vi "Measure.vi"(0 "Startfeld (T)":dbl=0.1, 1 "Zielfeld (T)":dbl=-0.1, 2 "Sweeprate (T/min)":dbl=0.05 min=0.0, 3 "Delay bei Null":bool=TRUE, 4 "Delay bei Max/Min":bool=TRUE, 5 "Delaytime bei Null (s)":u32=10, 6 "Anzahl Sweeps":u32=2, 7 "Deviation":u16(ring) items=["Normal", "Deviation"], 8 "Backsweep":bool=TRUE, 9 "Messmodus":u16(ring) items=["Nanosiemens", "Dissipation-tan(delta)", "Series - KilOhms", "GigOhms", "Loss Vector"], 10 "to Zero":bool=TRUE, 11 "error in (no error)":errorcluster) -> (14 "Ausgabe-Cluster":T1, 19 "error out":errorcluster)   [LabVIEW 2009]
panel:
  in  "Stop bei Target":bool
  out "Data":bool
  out "Done":bool
  in  "Delaytime bei Max/Min (s)":u32=10
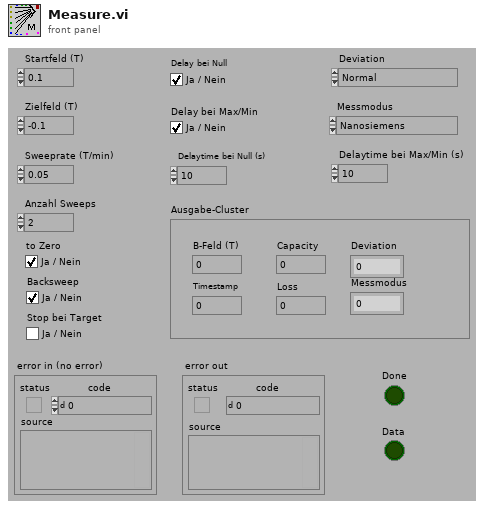
[diagram p1: front panel]
types:
  T1 = cluster{"B-Feld (T)":dbl, "Timestamp":dbl, "Capacity":dbl, "Loss":dbl, "Deviation":u16, "Messmodus":u16}
  T2 = cluster{"B-Feld":dbl, dbl, "capacitance":dbl, "loss":dbl, "Deviation":u16, "Messmodus":u16}
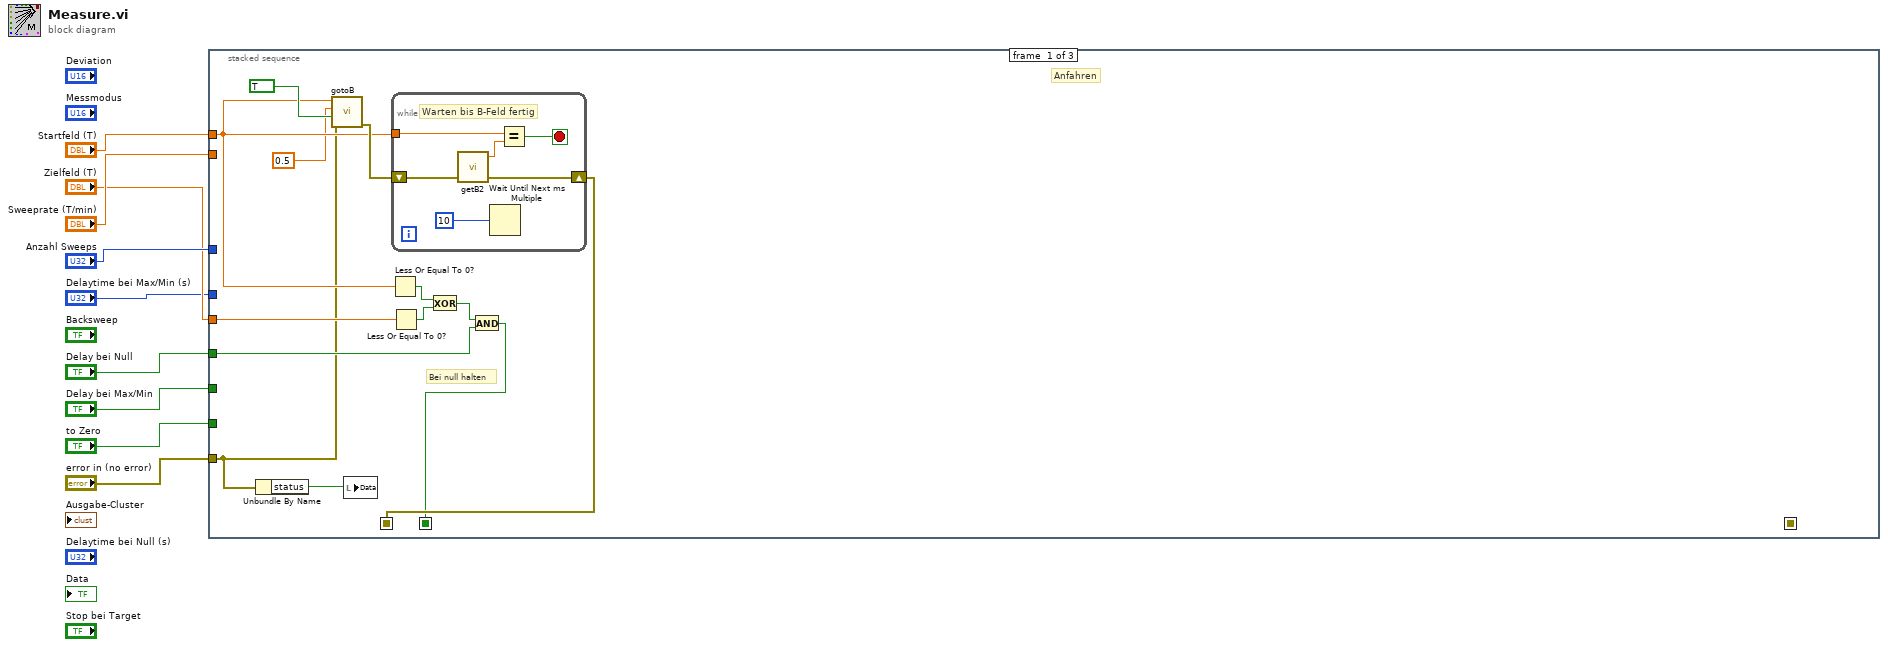
[diagram p0: block diagram]
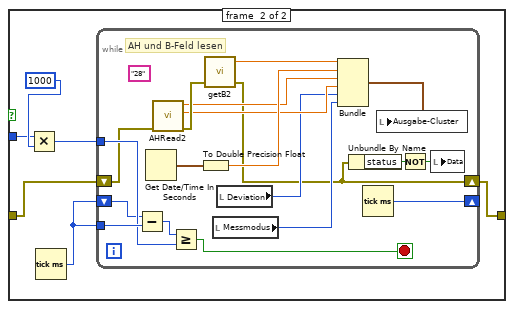
[diagram p3: hidden frame]
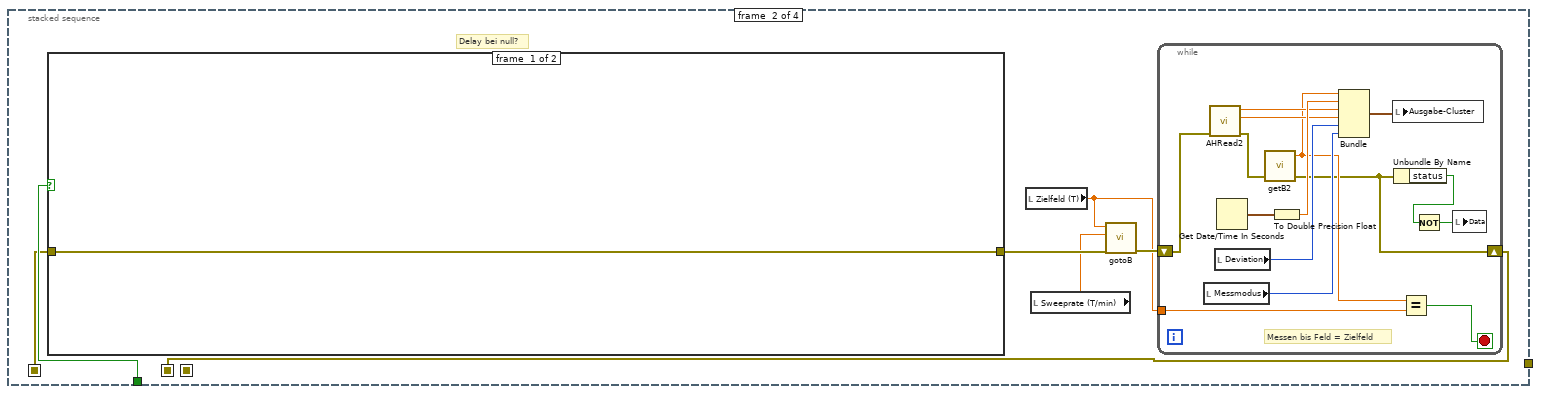
[diagram p4: hidden frame]
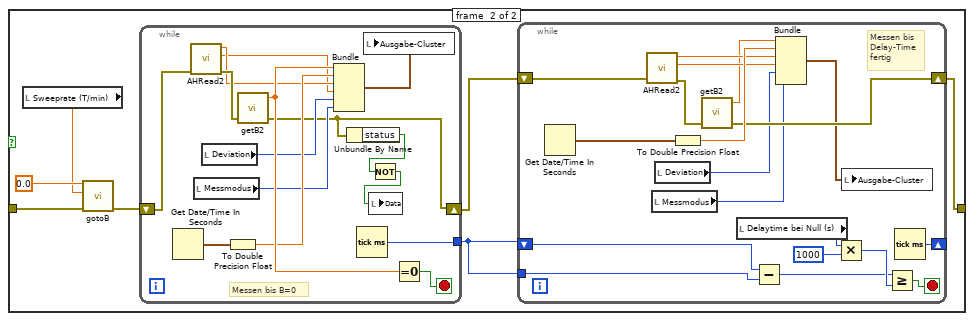
[diagram p5: hidden frame]
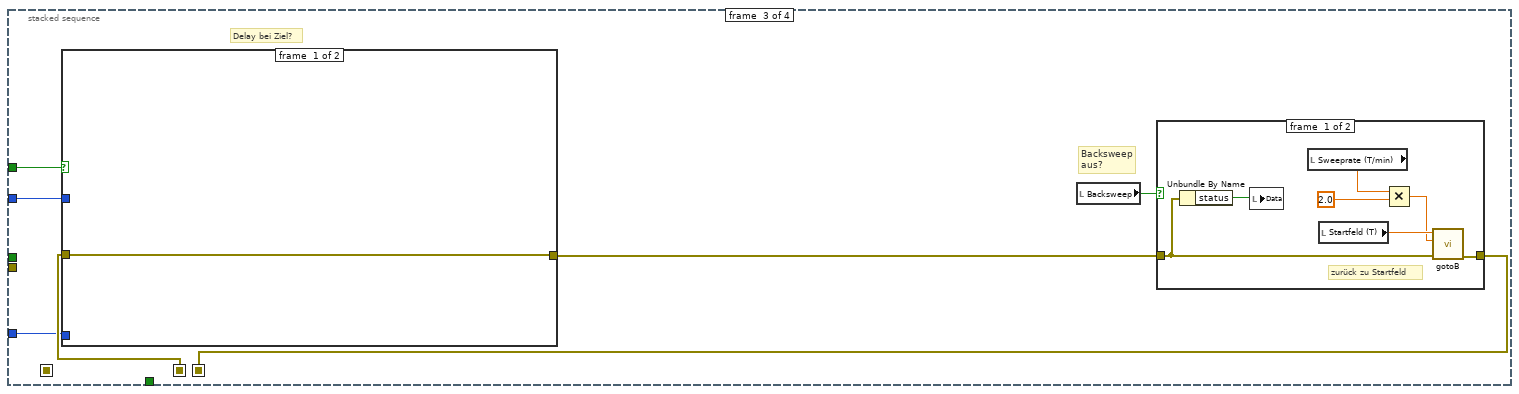
[diagram p6: hidden frame]
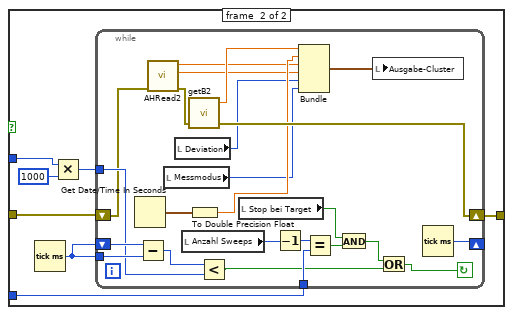
[diagram p8: hidden frame]
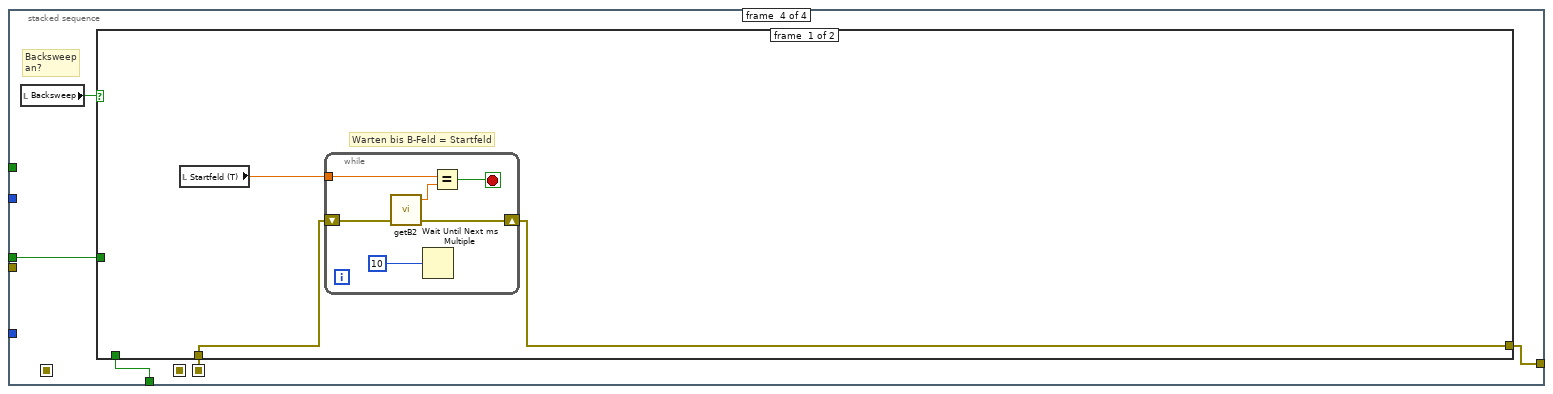
[diagram p9: hidden frame]
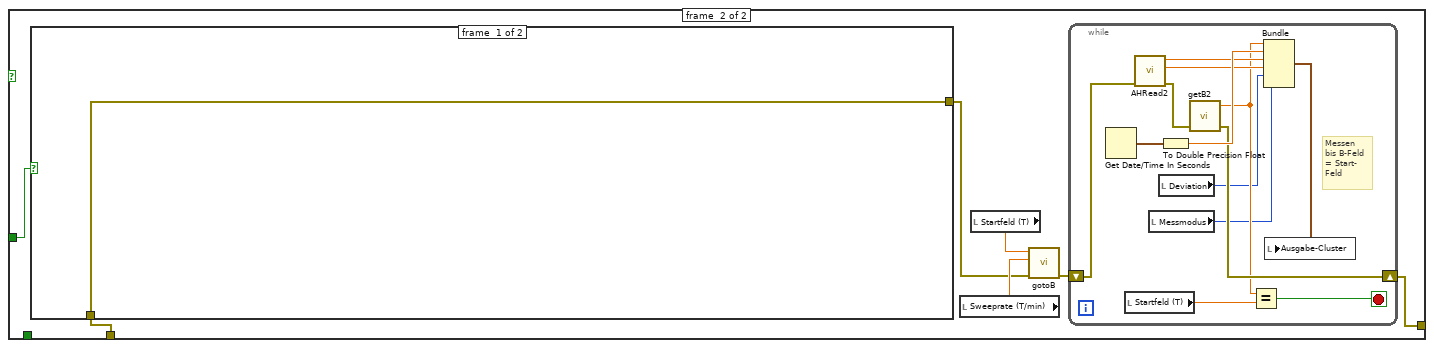
[diagram p10: hidden frame]
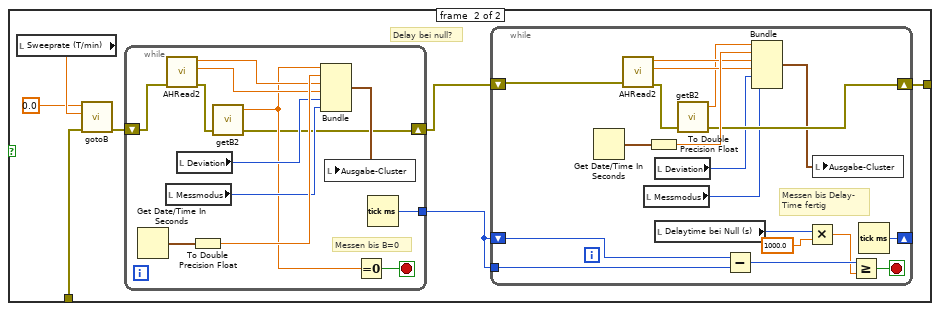
[diagram p11: hidden frame]
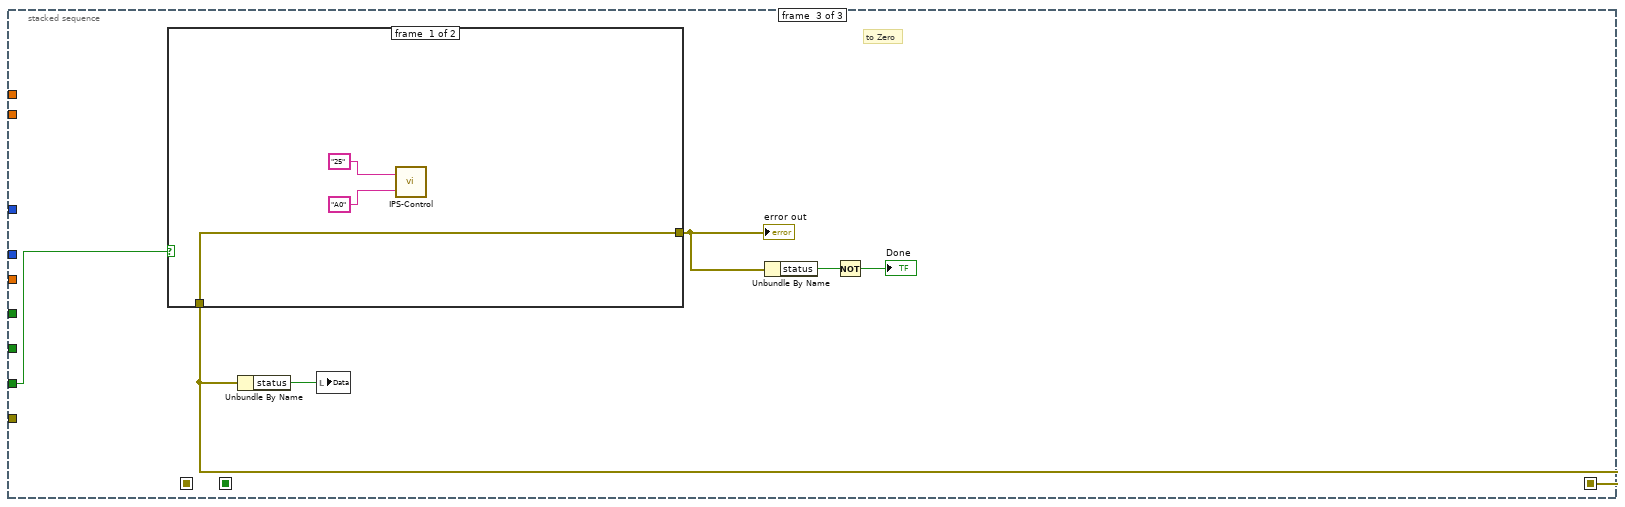
[diagram p12: hidden frame]
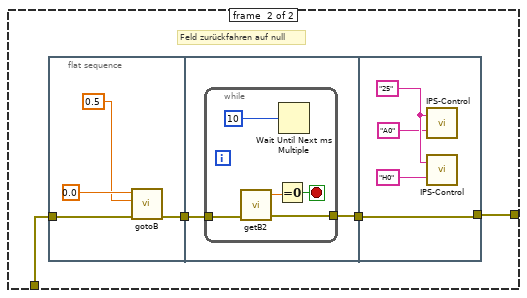
[diagram p13: hidden frame]
diagram:
  n1 = stacked-sequence {
    seq-local: [w20 _ _] -> [_ w36 _]
    seq-local: [w13 _ _] -> [_ w35 _]
    seq-local: [_ w30 _] -> [_ _ w261]
    tunnel: "Startfeld (T)" -> [w19 _ _]
    tunnel: "Sweeprate (T/min)" -> [_ w33 _]
    tunnel: "error in (no error)" -> [w12 _ _]
    tunnel: "Anzahl Sweeps" -> [_ w37 _]
    tunnel: "Zielfeld (T)" -> [w18 w34 _]
    tunnel: "Delay bei Null" -> [w14 w31 _]
    tunnel: "Delay bei Max/Min" -> [_ w32 _]
    tunnel: "to Zero" -> [_ _ w265]
    tunnel: "Delaytime bei Max/Min (s)" -> [_ w29 _]
    frame #0 {
      # "Bei null halten"
      # "Anfahren"
      n2 = Unbundle By Name(w12) -> ("status"=w11:bool)
      n3 = call "gotoB.vi"("error in (no error)"=w12, "Heater"=TRUE, "Sweeprate (T/min)"=0.5, "Target Field (T)"=w19) -> ("error out"=w21:errorcluster)  [unwired: 7 in]
      n4 = local write "Data"(w11) -> ()
      n5 = Less Or Equal To 0?(x=w19) -> (x <= 0?=w16:bool)
      n6 = Less Or Equal To 0?(x=w18) -> (x <= 0?=w17:bool)
      n7 = while {
        tunnel: w19 -> [w27]
        shift-right: [w25] -> w20
        shift-left: w21 -> [w26]
        stop <- w24 stop-if-true
        # "Warten bis B-Feld fertig"
        n8 = call "getB2.vi"("error in (no error)"=w26) -> ("error out"=w25:errorcluster, "B-Feld"=w28:dbl)  [unwired: 3 in]
        n9 = Wait Until Next ms Multiple(millisecond multiple=10) -> ()  [unwired: 1 out]
        n10 = Equal?(x=w27, y=w28) -> (x = y?=w24:bool)
      }
      n11 = Exclusive Or(1:w17, 2:w16) -> (0:w15:bool)
      n12 = And(x=w15, y=w14) -> (x .and. y?=w13:bool)
    }
    frame #1 {
      # "Wiederholung Anzahl Sweeps"
      # "Messung"
      n13 = for {
        N: w37 -> [_]
        shift-right: [w40] -> w30
        shift-left: w36 -> [w43]
        tunnel: w35 -> [w42]
        tunnel: w34 -> [_]
        tunnel: w33 -> [_]
        tunnel: w32 -> [w44]
        tunnel: w31 -> [w41]
        tunnel: w29 -> [w39]
        i -> [w38]
        n14 = stacked-sequence {
          seq-local: [w47 _ _ _] -> [_ w80 _ _]
          seq-local: [_ w75 _ _] -> [_ _ w144 _]
          seq-local: [_ _ w141 _] -> [_ _ _ w189]
          tunnel: w44 -> [w48 _ w145 _]
          tunnel: w43 -> [w45 _ _ _]
          tunnel: w42 -> [_ w81 _ w188]
          tunnel: w41 -> [_ _ _ w187]
          tunnel: [_ _ _ w186] -> w40
          tunnel: w39 -> [w46 _ w140 _]
          tunnel: w38 -> [_ _ w139 _]
          frame #0 {
            # "Delay bei Start?"
            n15 = case shown="True" w48 {
              tunnel: w45 -> [w49 w53]
              tunnel: [w49 w52] -> w47
              tunnel: w46 -> [_ w50]
              frame #0 {
              }
              frame #1 {
                n16 = Multiply(x=w50, y=1000) -> (x*y=w54:u32)
                n17 = Tick Count (ms)() -> (millisecond timer value=w51:u32)
                n18 = while {
                  tunnel: w51 -> [w74]
                  tunnel: w54 -> [w72]
                  shift-right: [w69] -> _
                  shift-left: w51 -> [w70]
                  shift-right: [w56] -> w52
                  shift-left: w53 -> [w68]
                  stop <- w71 stop-if-true
                  (unwired) "28"
                  # "AH und B-Feld lesen"
                  n19 = Subtract(x=w70, y=w74) -> (x-y=w73:u32)
                  n20 = Get Date/Time In Seconds() -> (seconds since 1Jan1904=w65:timestamp)
                  n21 = call "AHRead2.vi"("error in (no error)"=w68) -> ("error out"=w67:errorcluster, "loss"=w62:dbl, "capacitance"=w63:dbl)  [unwired: 7 in, 1 out]
                  n22 = Greater Or Equal?(x=w73, y=w72) -> (x >= y?=w71:bool)
                  n23 = To Double Precision Float(number=w65) -> (double precision float=w64:dbl)
                  n24 = call "getB2.vi"("error in (no error)"=w67) -> ("error out"=w56:errorcluster, "B-Feld"=w66:dbl)  [unwired: 3 in]
                  n25 = local read "Messmodus"() -> (w60:u16)
                  n26 = local read "Deviation"() -> (w61:u16)
                  n27 = Bundle("B-Feld"=w66, w64, "capacitance"=w63, "loss"=w62, "Deviation"=w61, "Messmodus"=w60) -> (w59:T2)  [unwired: 1 in]
                  n28 = Unbundle By Name(w56) -> ("status"=w57:bool)
                  n29 = Tick Count (ms)() -> (millisecond timer value=w69:u32)
                  n30 = local write "Ausgabe-Cluster"(w59) -> ()
                  n31 = Not(x=w57) -> (.not. x?=w58:bool)
                  n32 = local write "Data"(w58) -> ()
                }
              }
            }
          }
          frame #1 {
            # "Delay bei null?"
            n33 = case shown="True" w81 {
              tunnel: w80 -> [w97 w104]
              tunnel: [w97 w99] -> w79
              frame #0 {
              }
              frame #1 {
                n34 = local read "Sweeprate (T/min)"() -> (w102:dbl)
                n35 = call "gotoB.vi"("error in (no error)"=w104, "Sweeprate (T/min)"=w102, "Target Field (T)"=0.0) -> ("error out"=w101:errorcluster)  [unwired: 8 in]
                n36 = while {
                  shift-right: [w126] -> w100
                  shift-left: w101 -> [w136]
                  tunnel: [w127] -> w98
                  stop <- w138 stop-if-true
                  # "Messen bis B=0"
                  n37 = Get Date/Time In Seconds() -> (seconds since 1Jan1904=w134:timestamp)
                  n38 = call "AHRead2.vi"("error in (no error)"=w136) -> ("error out"=w137:errorcluster, "loss"=w131:dbl, "capacitance"=w132:dbl)  [unwired: 7 in, 1 out]
                  n39 = local read "Messmodus"() -> (w129:u16)
                  n40 = local read "Deviation"() -> (w130:u16)
                  n41 = To Double Precision Float(number=w134) -> (double precision float=w133:dbl)
                  n42 = call "getB2.vi"("error in (no error)"=w137) -> ("error out"=w126:errorcluster, "B-Feld"=w135:dbl)  [unwired: 3 in]
                  n43 = Bundle("B-Feld"=w135, w133, "capacitance"=w132, "loss"=w131, "Deviation"=w130, "Messmodus"=w129) -> (w128:T2)  [unwired: 1 in]
                  n44 = Unbundle By Name(w126) -> ("status"=w125:bool)
                  n45 = Tick Count (ms)() -> (millisecond timer value=w127:u32)
                  n46 = local write "Ausgabe-Cluster"(w128) -> ()
                  n47 = Not(x=w125) -> (.not. x?=w124:bool)
                  n48 = local write "Data"(w124) -> ()
                  n49 = Equal To 0?(x=w135) -> (x = 0?=w138:bool)
                }
                n50 = while {
                  shift-right: [w123] -> _
                  shift-left: w98 -> [w118]
                  tunnel: w98 -> [w119]
                  shift-right: [w109] -> w99
                  shift-left: w100 -> [w110]
                  stop <- w122 stop-if-true
                  # "Messen bis\nDelay-Time\nfertig"
                  n51 = Get Date/Time In Seconds() -> (seconds since 1Jan1904=w114:timestamp)
                  n52 = call "AHRead2.vi"("error in (no error)"=w110) -> ("error out"=w115:errorcluster, "loss"=w111:dbl, "capacitance"=w112:dbl)  [unwired: 7 in, 1 out]
                  n53 = local read "Messmodus"() -> (w107:u16)
                  n54 = local read "Deviation"() -> (w108:u16)
                  n55 = To Double Precision Float(number=w114) -> (double precision float=w113:dbl)
                  n56 = call "getB2.vi"("error in (no error)"=w115) -> ("error out"=w109:errorcluster, "B-Feld"=w106:dbl)  [unwired: 3 in]
                  n57 = local read "Delaytime bei Null (s)"() -> (w121:u32)
                  n58 = Subtract(x=w118, y=w119) -> (x-y=w116:u32)
                  n59 = Bundle("B-Feld"=w106, w113, "capacitance"=w112, "loss"=w111, "Deviation"=w108, "Messmodus"=w107) -> (w105:T2)  [unwired: 1 in]
                  n60 = Multiply(x=w121, y=u32 1000) -> (x*y=w117:u32)
                  n61 = local write "Ausgabe-Cluster"(w105) -> ()
                  n62 = Greater Or Equal?(x=w116, y=w117) -> (x >= y?=w122:bool)
                  n63 = Tick Count (ms)() -> (millisecond timer value=w123:u32)
                }
              }
            }
            n64 = local read "Zielfeld (T)"() -> (w76:dbl)
            n65 = local read "Sweeprate (T/min)"() -> (w78:dbl)
            n66 = call "gotoB.vi"("error in (no error)"=w79, "Sweeprate (T/min)"=w78, "Target Field (T)"=w76) -> ("error out"=w77:errorcluster)  [unwired: 8 in]
            n67 = while {
              shift-right: [w84] -> w75
              shift-left: w77 -> [w96]
              tunnel: w76 -> [w87]
              stop <- w85 stop-if-true
              # "Messen bis Feld = Zielfeld"
              n68 = local read "Messmodus"() -> (w89:u16)
              n69 = call "AHRead2.vi"("error in (no error)"=w96) -> ("error out"=w95:errorcluster, "loss"=w91:dbl, "capacitance"=w92:dbl)  [unwired: 7 in, 1 out]
              n70 = local read "Deviation"() -> (w90:u16)
              n71 = Get Date/Time In Seconds() -> (seconds since 1Jan1904=w94:timestamp)
              n72 = call "getB2.vi"("error in (no error)"=w95) -> ("error out"=w84:errorcluster, "B-Feld"=w86:dbl)  [unwired: 3 in]
              n73 = To Double Precision Float(number=w94) -> (double precision float=w93:dbl)
              n74 = Bundle("B-Feld"=w86, w93, "capacitance"=w92, "loss"=w91, "Deviation"=w90, "Messmodus"=w89) -> (w88:T2)  [unwired: 1 in]
              n75 = local write "Ausgabe-Cluster"(w88) -> ()
              n76 = Unbundle By Name(w84) -> ("status"=w82:bool)
              n77 = Equal?(x=w86, y=w87) -> (x = y?=w85:bool)
              n78 = Not(x=w82) -> (.not. x?=w83:bool)
              n79 = local write "Data"(w83) -> ()
            }
          }
          frame #2 {
            # "Backsweep\naus?"
            # "Delay bei Ziel?"
            n80 = case shown="True" w145 {
              tunnel: w144 -> [w154 w159]
              tunnel: [w154 w158] -> w142
              tunnel: w140 -> [_ w156]
              tunnel: w139 -> [_ w155]
              frame #0 {
              }
              frame #1 {
                n81 = Tick Count (ms)() -> (millisecond timer value=w157:u32)
                n82 = Multiply(x=w156, y=u32 1000) -> (x*y=w160:u32)
                n83 = while {
                  shift-right: [w185] -> _
                  shift-left: w157 -> [w184]
                  tunnel: w157 -> [w183]
                  tunnel: w160 -> [w182]
                  shift-right: [w178] -> w158
                  shift-left: w159 -> [w179]
                  tunnel: w155 -> [w169]
                  stop <- w165 continue-if-true
                  n84 = Get Date/Time In Seconds() -> (seconds since 1Jan1904=w176:timestamp)
                  n85 = Subtract(x=w184, y=w183) -> (x-y=w181:u32)
                  n86 = call "AHRead2.vi"("error in (no error)"=w179) -> ("error out"=w180:errorcluster, "loss"=w173:dbl, "capacitance"=w174:dbl)  [unwired: 7 in, 1 out]
                  n87 = local read "Messmodus"() -> (w171:u16)
                  n88 = local read "Deviation"() -> (w172:u16)
                  n89 = local read "Anzahl Sweeps"() -> (w163:u32)
                  n90 = call "getB2.vi"("error in (no error)"=w180) -> ("error out"=w178:errorcluster, "B-Feld"=w177:dbl)  [unwired: 3 in]
                  n91 = To Double Precision Float(number=w176) -> (double precision float=w175:dbl)
                  n92 = Less?(x=w181, y=w182) -> (x < y?=w164:bool)
                  n93 = local read "Stop bei Target"() -> (w167:bool)
                  n94 = Decrement(x=w163) -> (x-1=w162:u32)
                  n95 = Bundle("B-Feld"=w177, w175, "capacitance"=w174, "loss"=w173, "Deviation"=w172, "Messmodus"=w171) -> (w170:T2)  [unwired: 1 in]
                  n96 = Equal?(x=w162, y=w169) -> (x = y?=w168:bool)
                  n97 = And(x=w167, y=w168) -> (x .and. y?=w166:bool)
                  n98 = local write "Ausgabe-Cluster"(w170) -> ()
                  n99 = Or(x=w166, y=w164) -> (x .or. y?=w165:bool)
                  n100 = Tick Count (ms)() -> (millisecond timer value=w185:u32)
                }
              }
            }
            n101 = local read "Backsweep"() -> (w143:bool)
            n102 = case shown="False" w143 {
              tunnel: w142 -> [w147 w153]
              tunnel: [w151 w153] -> w141
              frame #0 {
                # "zurück zu Startfeld"
                n103 = Unbundle By Name(w147) -> ("status"=w146:bool)
                n104 = local write "Data"(w146) -> ()
                n105 = local read "Sweeprate (T/min)"() -> (w150:dbl)
                n106 = local read "Startfeld (T)"() -> (w152:dbl)
                n107 = Multiply(x=w150, y=2.0) -> (x*y=w148:dbl)
                n108 = call "gotoB.vi"("error in (no error)"=w147, "Sweeprate (T/min)"=w148, "Target Field (T)"=w152) -> ("error out"=w151:errorcluster)  [unwired: 8 in]
              }
              frame #1 {
              }
            }
          }
          frame #3 {
            # "Backsweep\nan?"
            n109 = local read "Backsweep"() -> (w190:bool)
            n110 = case shown="True" w190 {
              tunnel: w189 -> [w192 w206]
              tunnel: [w191 w200] -> w186
              tunnel: w188 -> [_ _]
              tunnel: w187 -> [_ w205]
              frame #0 {
                # "Warten bis B-Feld = Startfeld"
                n111 = local read "Startfeld (T)"() -> (w193:dbl)
                n112 = while {
                  tunnel: w193 -> [w198]
                  shift-right: [w196] -> w191
                  shift-left: w192 -> [w197]
                  stop <- w195 stop-if-true
                  n113 = call "getB2.vi"("error in (no error)"=w197) -> ("error out"=w196:errorcluster, "B-Feld"=w199:dbl)  [unwired: 3 in]
                  n114 = Wait Until Next ms Multiple(millisecond multiple=10) -> ()  [unwired: 1 out]
                  n115 = Equal?(x=w198, y=w199) -> (x = y?=w195:bool)
                }
              }
              frame #1 {
                n116 = case shown="True" w205 {
                  tunnel: w206 -> [w220 w224]
                  tunnel: [w220 w222] -> w202
                  frame #0 {
                  }
                  frame #1 {
                    # "Delay bei null?"
                    n117 = local read "Sweeprate (T/min)"() -> (w227:dbl)
                    n118 = call "gotoB.vi"("error in (no error)"=w224, "Sweeprate (T/min)"=w227, "Target Field (T)"=0.0) -> ("error out"=w225:errorcluster)  [unwired: 8 in]
                    n119 = while {
                      shift-right: [w248] -> w223
                      shift-left: w225 -> [w255]
                      tunnel: [w247] -> w221
                      stop <- w258 stop-if-true
                      # "Messen bis B=0"
                      n120 = Get Date/Time In Seconds() -> (seconds since 1Jan1904=w256:timestamp)
                      n121 = local read "Messmodus"() -> (w250:u16)
                      n122 = call "AHRead2.vi"("error in (no error)"=w255) -> ("error out"=w259:errorcluster, "loss"=w252:dbl, "capacitance"=w253:dbl)  [unwired: 7 in, 1 out]
                      n123 = local read "Deviation"() -> (w251:u16)
                      n124 = To Double Precision Float(number=w256) -> (double precision float=w254:dbl)
                      n125 = call "getB2.vi"("error in (no error)"=w259) -> ("error out"=w248:errorcluster, "B-Feld"=w249:dbl)  [unwired: 3 in]
                      n126 = Bundle("B-Feld"=w249, w254, "capacitance"=w253, "loss"=w252, "Deviation"=w251, "Messmodus"=w250) -> (w257:T2)  [unwired: 1 in]
                      n127 = local write "Ausgabe-Cluster"(w257) -> ()
                      n128 = Equal To 0?(x=w249) -> (x = 0?=w258:bool)
                      n129 = Tick Count (ms)() -> (millisecond timer value=w247:u32)
                    }
                    n130 = while {
                      shift-right: [w242] -> _
                      shift-left: w221 -> [w243]
                      tunnel: w221 -> [w244]
                      shift-right: [w231] -> w222
                      shift-left: w223 -> [w232]
                      stop <- w239 stop-if-true
                      # "Messen bis Delay-\nTime fertig"
                      n131 = Get Date/Time In Seconds() -> (seconds since 1Jan1904=w237:timestamp)
                      n132 = call "AHRead2.vi"("error in (no error)"=w232) -> ("error out"=w238:errorcluster, "loss"=w234:dbl, "capacitance"=w235:dbl)  [unwired: 7 in, 1 out]
                      n133 = local read "Messmodus"() -> (w229:u16)
                      n134 = To Double Precision Float(number=w237) -> (double precision float=w236:dbl)
                      n135 = local read "Deviation"() -> (w230:u16)
                      n136 = local read "Delaytime bei Null (s)"() -> (w240:u32)
                      n137 = call "getB2.vi"("error in (no error)"=w238) -> ("error out"=w231:errorcluster, "B-Feld"=w233:dbl)  [unwired: 3 in]
                      n138 = Subtract(x=w243, y=w244) -> (x-y=w245:u32)
                      n139 = Bundle("B-Feld"=w233, w236, "capacitance"=w235, "loss"=w234, "Deviation"=w230, "Messmodus"=w229) -> (w228:T2)  [unwired: 1 in]
                      n140 = Multiply(x=w240, y=1000.0) -> (x*y=w241:dbl)
                      n141 = local write "Ausgabe-Cluster"(w228) -> ()
                      n142 = Greater Or Equal?(x=w245, y=w241) -> (x >= y?=w239:bool)
                      n143 = Tick Count (ms)() -> (millisecond timer value=w242:u32)
                    }
                  }
                }
                n144 = local read "Sweeprate (T/min)"() -> (w203:dbl)
                n145 = local read "Startfeld (T)"() -> (w204:dbl)
                n146 = call "gotoB.vi"("error in (no error)"=w202, "Sweeprate (T/min)"=w203, "Target Field (T)"=w204) -> ("error out"=w201:errorcluster)  [unwired: 8 in]
                n147 = while {
                  shift-right: [w213] -> w200
                  shift-left: w201 -> [w214]
                  stop <- w210 stop-if-true
                  # "Messen\nbis B-Feld\n= Start-\nFeld"
                  n148 = Get Date/Time In Seconds() -> (seconds since 1Jan1904=w218:timestamp)
                  n149 = local read "Startfeld (T)"() -> (w212:dbl)
                  n150 = call "AHRead2.vi"("error in (no error)"=w214) -> ("error out"=w219:errorcluster, "loss"=w215:dbl, "capacitance"=w216:dbl)  [unwired: 7 in, 1 out]
                  n151 = local read "Messmodus"() -> (w208:u16)
                  n152 = local read "Deviation"() -> (w209:u16)
                  n153 = To Double Precision Float(number=w218) -> (double precision float=w217:dbl)
                  n154 = call "getB2.vi"("error in (no error)"=w219) -> ("error out"=w213:errorcluster, "B-Feld"=w211:dbl)  [unwired: 3 in]
                  n155 = Equal?(x=w211, y=w212) -> (x = y?=w210:bool)
                  n156 = Bundle("B-Feld"=w211, w217, "capacitance"=w216, "loss"=w215, "Deviation"=w209, "Messmodus"=w208) -> (w207:T2)  [unwired: 1 in]
                  n157 = local write "Ausgabe-Cluster"(w207) -> ()
                }
              }
            }
          }
        }
      }
    }
    frame #2 {
      # "to Zero"
      n158 = case shown="True" w265 {
        tunnel: w261 -> [w268 w272]
        tunnel: [w268 w271] -> w262
        frame #0 {
          n159 = call "IPS-Control.vi"("Frage"="A0", "address string"="25") -> ()  [unwired: 1 out]
        }
        frame #1 {
          # "Feld zurückfahren auf null"
          n160 = flat-sequence {
            tunnel: w272 -> [w276]
            tunnel: [w274] -> w270
            tunnel: w270 -> [w278]
            tunnel: [w277] -> w269
            tunnel: w269 -> [w287]
            tunnel: [w287] -> w271
            frame #0 {
              n161 = call "gotoB.vi"("error in (no error)"=w276, "Sweeprate (T/min)"=0.5, "Target Field (T)"=0.0) -> ("error out"=w274:errorcluster)  [unwired: 8 in]
            }
            frame #1 {
              n162 = while {
                tunnel: w278 -> [w283]
                tunnel: [w280] -> w277
                stop <- w281 stop-if-true
                n163 = call "getB2.vi"("error in (no error)"=w283) -> ("error out"=w280:errorcluster, "B-Feld"=w282:dbl)  [unwired: 3 in]
                n164 = Equal To 0?(x=w282) -> (x = 0?=w281:bool)
                n165 = Wait Until Next ms Multiple(millisecond multiple=10) -> ()  [unwired: 1 out]
              }
            }
            frame #2 {
              w286 = "25"
              n166 = call "IPS-Control.vi"("Frage"="A0", "address string"=w286) -> ()  [unwired: 1 out]
              n167 = call "IPS-Control.vi"("Frage"="H0", "address string"=w286) -> ()  [unwired: 1 out]
            }
          }
        }
      }
      "error out" <- w262
      n168 = Unbundle By Name(w261) -> ("status"=w260:bool)
      n169 = local write "Data"(w260) -> ()
      n170 = Unbundle By Name(w262) -> ("status"=w263:bool)
      n171 = Not(x=w263) -> (.not. x?=→"Done":bool)
    }
  }
